vi "ICS425.vi"(0 "VISA resource name":refnum<visa-resource-name>="SETRA", 1 "Runtime Gather?":bool, 11 "Error In":errorcluster) -> (4 "Weight Output":dbl, 6 "Weight Output (string)":string, 15 "Error Out":errorcluster)   [LabVIEW 2018]
uses:
  Type Definitions/ICS245_Commands.ctl
panel:
  in  "?":enum32{"MAIN", "Configuration"}(tab)
  in  "Accept Reading":bool
  in  "Zero Button":bool
  in  "Read Scale":bool
  out "Stable Reading":bool
  in  "Weight":dbl
  out "Read Buffer":string
  out "concatenated input string":string
  out "concatenated input string 2":string
  # "ICS 425 Scale Reading"
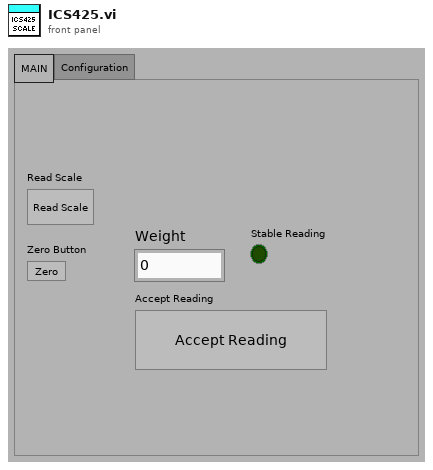
[diagram p1: front panel]
types:
  T1 = typedef "ICS245_Commands.ctl" = string
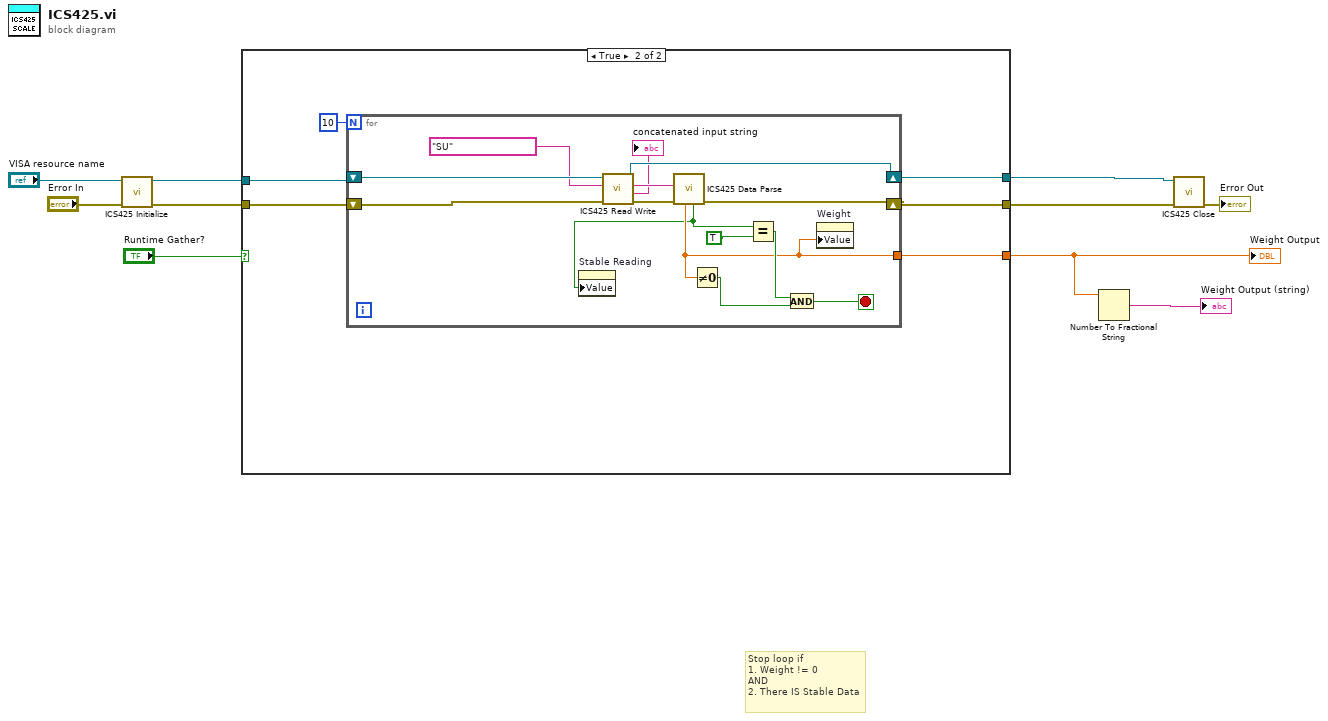
[diagram p0: block diagram]
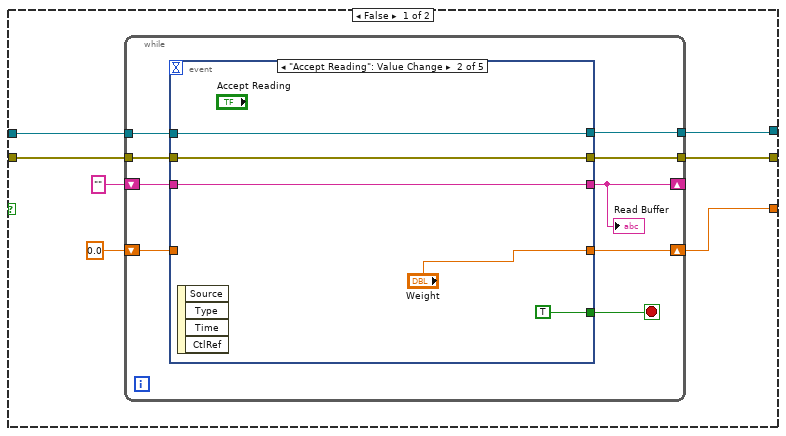
[diagram p2: hidden frame]
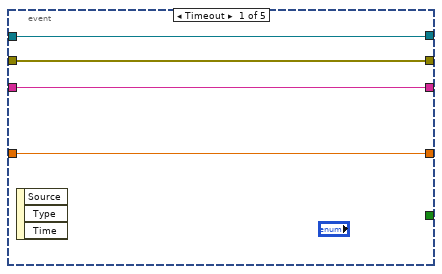
[diagram p3: hidden frame]
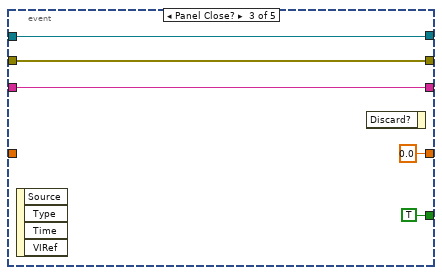
[diagram p4: hidden frame]
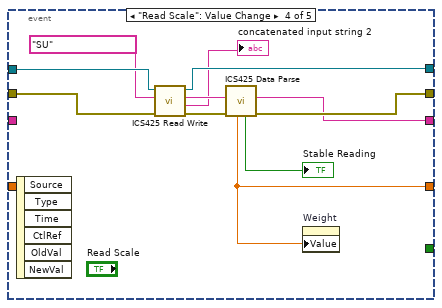
[diagram p5: hidden frame]
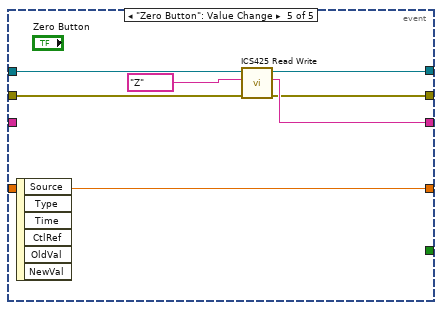
[diagram p6: hidden frame]
diagram:
  # "Stop loop if\n1. Weight != 0\nAND \n2. There IS Stable Data"
  n1 = call "ICS425 Initialize.vi"("Error In"="Error In", "VISA Refnum in"="VISA resource name") -> ("Error Out"=w7:errorcluster, "VISA Refnum out"=w8:refnum<visa-resource-name>)  [unwired: 8 in]
  n2 = case shown="True" "Runtime Gather?" {
    tunnel: w8 -> [w17 w64]
    tunnel: w7 -> [w15 w63]
    tunnel: [w16 w62] -> w5
    tunnel: [w14 w61] -> w4
    tunnel: [w13 w60] -> w1
    frame False {
      n3 = while {
        tunnel: w17 -> [w26]
        tunnel: [w25] -> w16
        tunnel: w15 -> [w24]
        tunnel: [w23] -> w14
        shift-right: [w22] -> w13
        shift-left: 0.0 ("Weight") -> [w21]
        shift-right: [w19] -> _
        shift-left: "" -> [w20]
        stop <- w18 stop-if-true
        n4 = event shown="[1] \"Accept Reading\": Value Change" {
          selector: _ -> [_ _ _ _ _]
          dyn-events: _ -> [_ _ _ _ _]
          timeout: _ -> [_ _ _ _ _]
          tunnel: w26 -> [w30 w33 w40 w48 w57]
          tunnel: [w30 w33 w40 w49 w53] -> w25
          tunnel: w24 -> [w29 w32 w39 w46 w56]
          tunnel: [w29 w32 w39 w45 w54] -> w23
          tunnel: w21 -> [w28 _ _ _ w52]
          tunnel: [w28 "Weight" 0.0 ("Weight") w41 w52] -> w22
          tunnel: w20 -> [w27 w35 w38 _ _]
          tunnel: [w27 w35 w38 w42 w55] -> w19
          tunnel: [_ TRUE TRUE _ _] -> w18
          event Timeout {
            n5 = event-data() -> ()  [unwired: 1 in, 3 out]
          }
          event "Accept Reading": Value Change {
            n6 = event-data() -> ()  [unwired: 1 in, 4 out]
          }
          event Panel Close? {
            n7 = event-data() -> ()  [unwired: 1 in, 4 out]
            n8 = event-data() -> ()  [unwired: 2 in, 1 out]
          }
          event "Read Scale": Value Change {
            n9 = event-data() -> ()  [unwired: 1 in, 6 out]
            n10 = call "ICS425 Read Write.vi"("Error In"=w46, "Cmd"=T1 "SU" ("ICS245 Commands"), "VISA (Input)"=w48) -> ("Error Out"=w50:errorcluster, "concatenated input string"=→"concatenated input string 2":string, "read buffer"=w51:string, "VISA Refnum (Output)"=w49:refnum<visa-resource-name>)  [unwired: 5 in]
            n11 = call "ICS425 Data Parse.vi"("Error In"=w50, "Input Data"=w51) -> ("Error Out"=w45:errorcluster, "Output Data"=w42:string, "Data & Stability"=→"Stable Reading":bool, "Weight"=w41:dbl)  [unwired: 6 in]
            n12 = property on="Weight" class="DigNum (strict)"("Value"=w41) -> ()  [unwired: 2 in, 2 out]
          }
          event "Zero Button": Value Change {
            n13 = event-data() -> ()  [unwired: 1 in, 6 out]
            n14 = call "ICS425 Read Write.vi"("Error In"=w56, "Cmd"=T1 "Z" ("ICS245 Commands"), "VISA (Input)"=w57) -> ("Error Out"=w54:errorcluster, "read buffer"=w55:string, "VISA Refnum (Output)"=w53:refnum<visa-resource-name>)  [unwired: 5 in, 1 out]
          }
        }
        "Read Buffer" <- w19
      }
    }
    frame True {
      n15 = for {
        N: 10 -> [_]
        tunnel: [w66] -> w60
        shift-right: [w76] -> w62
        shift-left: w64 -> [w78]
        shift-right: [w73] -> w61
        shift-left: w63 -> [w77]
        stop <- w69 stop-if-true
        n16 = call "ICS425 Read Write.vi"("Error In"=w77, "Cmd"=T1 "SU" ("ICS245 Commands"), "VISA (Input)"=w78) -> ("Error Out"=w74:errorcluster, "concatenated input string"=→"concatenated input string":string, "read buffer"=w75:string, "VISA Refnum (Output)"=w76:refnum<visa-resource-name>)  [unwired: 5 in]
        n17 = call "ICS425 Data Parse.vi"("Error In"=w74, "Input Data"=w75) -> ("Error Out"=w73:errorcluster, "Data & Stability"=w65:bool, "Weight"=w66:dbl)  [unwired: 6 in, 1 out]
        n18 = property on="Stable Reading" class="Bool (strict)"("Value"=w65) -> ()  [unwired: 2 in, 2 out]
        n19 = Not Equal To 0?(x=w66) -> (x != 0?=w72:bool)
        n20 = Equal?(x=w65, y=TRUE) -> (x = y?=w70:bool)
        n21 = And(x=w70, y=w72) -> (x .and. y?=w69:bool)
        n22 = property on="Weight" class="DigNum (strict)"("Value"=w66) -> ()  [unwired: 2 in, 2 out]
      }
    }
  }
  "Weight Output" <- w1
  n23 = Number To Fractional String(number=w1) -> (F-format string=→"Weight Output (string)":string)  [unwired: 3 in]
  n24 = call "ICS425 Close.vi"("Error In"=w4, "VISA Refnum in"=w5) -> ("Error Out"=→"Error Out":errorcluster)  [unwired: 9 in]
